vi "21-sub.vi"(3 "Number":i32=5) -> (1 "Amicable Divisors Sum":i32)   [LabVIEW 2021]
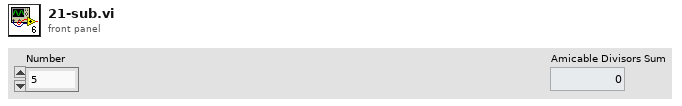
[diagram p1: front panel]
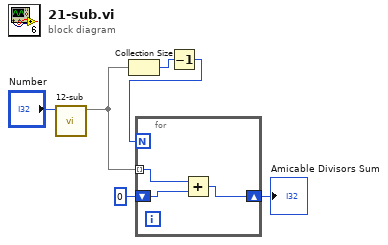
[diagram p0: block diagram]
diagram:
  n1 = call "12-sub.vi"("Number"="Number") -> ("Divisors"=w5:set{i32})  [unwired: 9 in, 1 out]
  n2 = Collection Size(1:w5) -> (0:w4:i32)
  n3 = Decrement(x=w4) -> (x-1=w3:i32)
  n4 = for {
    N: w3 -> [_]
    tunnel: w5 -> [w9] mode=indexing
    shift-right: [w7] -> w1
    shift-left: 0 -> [w8]
    n5 = Add(x=w9, y=w8) -> (x+y=w7:i32)
  }
  "Amicable Divisors Sum" <- w1
